vi "On Install of JSONtext.vi"() -> ()   [LabVIEW 2020]
uses:
  <vilib>/Palette API/Palette Menu/Public Type Define/Palette type.ctl
  <vilib>/Palette API/Palette Menu/Public Type Define/Item.ctl
  <vilib>/Palette API/Palette Menu/Palette Menu.lvlib
panel:
  out "error out":errorcluster
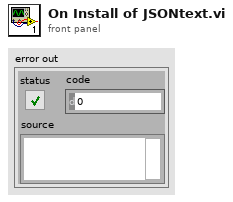
[diagram p1: front panel]
types:
  T1 = typedef "Palette Menu.lvlib/Palette type.ctl" = i32
  T2 = typedef "Palette Menu.lvlib/Palette Data.ctl" = cluster{"display name":string, "view format":T3, "palette width":i16, "items":T4, "256 color icon":picture, "B&W color icon":picture, "help information":T6, "palette description":string, "synchronize information":T7}
  T3 = typedef "Palette Menu.lvlib/View Format.ctl" = u16
  T4 = typedef "Palette Menu.lvlib/Items.ctl" = T5[]
  T5 = typedef "Palette Menu.lvlib/Item.ctl" = cluster{"item path":path, "library path":path, "use default lvlib palette":bool, "short name":string, "place VI contents":bool, "hide synchronized item":bool, "reserve spot for synch item":bool, "configure when placing VI contents":bool}
  T6 = typedef "Palette Menu.lvlib/Help Info.ctl" = cluster{"help tag":string, "help file path ":path}
  T7 = typedef "Palette Menu.lvlib/Synchronize Info.ctl" = cluster{"synchronize with directory":bool, "synchronize directory path":path}
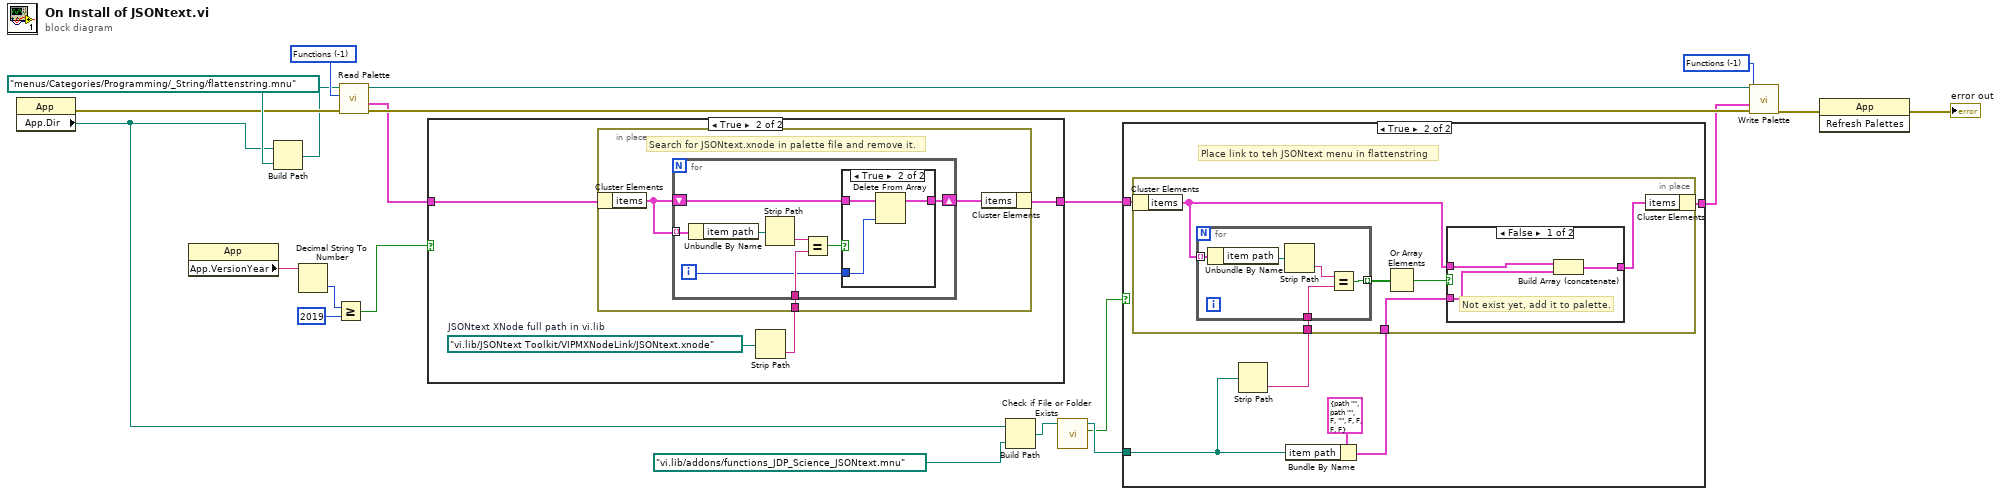
[diagram p0: block diagram]
diagram:
  w12 = T1 -1 items=["Functions"=-1, "Controls"=-2] ("palette type")
  w17 = T1 -1 items=["Functions"=-1, "Controls"=-2] ("palette type")
  n1 = property class="App"() -> (error out=w11:errorcluster, "App.Dir"=w1:path)  [unwired: 2 in, 1 out]
  n2 = property class="App"() -> ("App.VersionYear"=w19:string)  [unwired: 2 in, 2 out]
  n3 = Build Path(base path=w1, name or relative path=path "menus/Categories/Programming/_String/flattenstring.mnu") -> (appended path=w6:path)
  n4 = Decimal String To Number(string=w19) -> (number=w21:i32)  [unwired: 2 in, 1 out]
  n5 = Greater Or Equal?(x=w21, y=2019) -> (x >= y?=w18:bool)
  n6 = call <vilib>:"Read Palette.vi"("error in (no error)"=w11, "palette type"=w17, "palette path"=w6) -> ("error out"=w10:errorcluster, "palette data"=w9:T2, "duplicate palette path"=w15:path)  [unwired: 1 in, 5 out]
  n7 = case shown="True" w18 {
    tunnel: w9 -> [w22 w24]
    tunnel: [w22 w23] -> w8
    frame False {
    }
    frame True {
      w26 = path "vi.lib/JSONtext Toolkit/VIPMXNodeLink/JSONtext.xnode"  # JSONtext XNode full path in vi.lib
      n8 = Strip Path(path=w26) -> (name=w25:string)  [unwired: 1 out]
      n9 = in-place {
        in-place-border: w25 -> [w29]
        # "Search for JSONtext.xnode in palette file and remove it."
        n10 = in-place-cluster #1(w24) -> ("items"=w28:T4)
        n11 = for {
          tunnel: w28 -> [w37] mode=indexing
          tunnel: w29 -> [w34]
          shift-right: [w30] -> w27
          shift-left: w28 -> [w32]
          i -> [w31]
          n12 = Unbundle By Name(w37) -> ("item path"=w36:path)
          n13 = Strip Path(path=w36) -> (name=w35:string)  [unwired: 1 out]
          n14 = Equal?(x=w35, y=w34) -> (x = y?=w33:bool)
          n15 = case shown="True" w33 {
            tunnel: w32 -> [w38 w40]
            tunnel: w31 -> [_ w41]
            tunnel: [w38 w39] -> w30
            frame False {
            }
            frame True {
              n16 = Delete From Array(array=w40, index=w41) -> (array with subset deleted=w39:T4)  [unwired: 1 in, 1 out]
            }
          }
        }
        n17 = in-place-cluster #1("items"=w27) -> (w23:T2)
      }
    }
  }
  n18 = Build Path(base path=w1, name or relative path=path "vi.lib/addons/functions_JDP_Science_JSONtext.mnu") -> (appended path=w5:path)
  n19 = call <vilib>:"Check if File or Folder Exists.vi"("path"=w5) -> ("file or folder exists?"=w2:bool, "dup path"=w4:path)  [unwired: 8 in, 1 out]
  n20 = case shown="True" w2 {
    tunnel: w8 -> [w42 w48]
    tunnel: w4 -> [_ w43]
    tunnel: [w42 w45] -> w3
    frame False {
    }
    frame True {
      # "Place link to teh JSONtext menu in flattenstring"
      n21 = Strip Path(path=w43) -> (name=w44:string)  [unwired: 1 out]
      n22 = Bundle By Name(cluster=T5 {"item path"=path "", "library path"=path "", "use default lvlib palette"=FALSE, "short name"="", "place VI contents"=FALSE, "hide synchronized item"=FALSE, "reserve spot for synch item"=FALSE, "configure when placing VI contents"=FALSE} ("Items"), "item path"=w43) -> (w46:T5)
      n23 = in-place {
        in-place-border: w44 -> [w54]
        in-place-border: w46 -> [w49]
        n24 = in-place-cluster #2(w48) -> ("items"=w50:T4)
        n25 = for {
          tunnel: w50 -> [w63] mode=indexing
          tunnel: w54 -> [w60]
          tunnel: [w59] -> w53 mode=indexing
          n26 = Unbundle By Name(w63) -> ("item path"=w62:path)
          n27 = Strip Path(path=w62) -> (name=w61:string)  [unwired: 1 out]
          n28 = Equal?(x=w61, y=w60) -> (x = y?=w59:bool)
        }
        n29 = Or Array Elements(Boolean array=w53) -> (logical OR=w52:bool)
        n30 = case shown="False" w52 {
          tunnel: w49 -> [w57 _]
          tunnel: [w56 w58] -> w51
          tunnel: w50 -> [w55 w58]
          frame False {
            # "Not exist yet, add it to palette."
            n31 = Build Array (concatenate)(w55, w57) -> (w56:T4)
          }
          frame True {
            # "Alreay exists on palette,\ndo nothing."
          }
        }
        n32 = in-place-cluster #2("items"=w51) -> (w45:T2)
      }
    }
  }
  n33 = call <vilib>:"Write Palette.vi"("error in (no error)"=w10, "palette data"=w3, "palette type"=w12, "palette path"=w15) -> ("error out"=w13:errorcluster)  [unwired: 1 in, 6 out]
  n34 = invoke class="App" method="Refresh Palettes"(error in=w13) -> (error out=→"error out":errorcluster)  [unwired: 2 in, 2 out]
